vi "MakeEngine.vi"(8 "error in (no error)":errorcluster, 11 "ClassicType in":refnum<class "ClassicType.lvclass">) -> (0 "error out":errorcluster, 3 "ClassicType out":refnum<class "ClassicType.lvclass">)   [LabVIEW 2021, in "ClassicType.lvclass"]
uses:
  ClassicType.lvclass
  C:/Users/chrismadlax/Documents/LabVIEW Data/Project/OOP/GeneralCar/GeneralCar.lvclass
  GeneralCar/GeneralCar.lvclass/GeneralCar.ctl
  GeneralCar/GeneralCar.lvclass
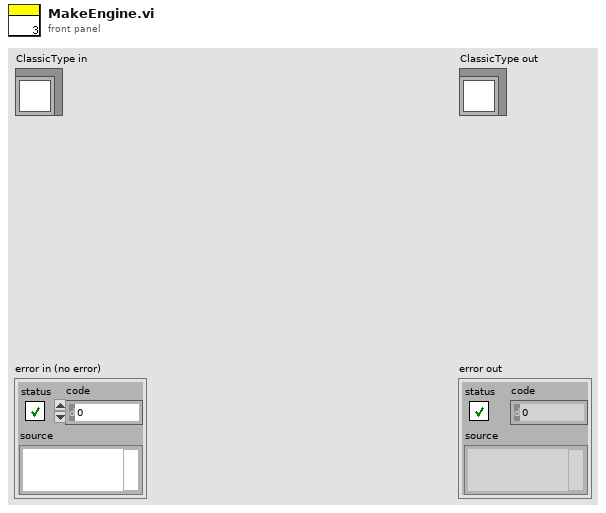
[diagram p1: front panel]
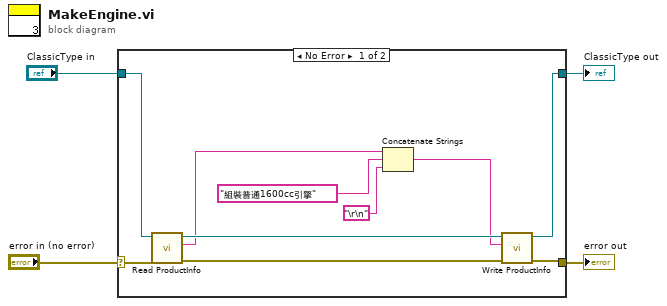
[diagram p0: block diagram]
diagram:
  n1 = case shown="No Error" "error in (no error)" {
    selector: "error in (no error)" -> [w7 w16]
    tunnel: [w6 w16] -> w4
    tunnel: [w5 w15] -> w3
    tunnel: "ClassicType in" -> [w8 w15]
    frame No Error {
      n2 = call "Read ProductInfo.vi"("error in (no error)"=w7, "GeneralCar in"=w8) -> ("error out"=w14:errorcluster, "ProductInfo"=w10:string, "GeneralCar out"=w13:refnum<class "ClassicType.lvclass">)  [unwired: 7 in]
      n3 = Concatenate Strings(w10, "組裝普通1600cc引擎" ("string"), "\r\n") -> (w9:string)
      n4 = call "Write ProductInfo.vi"("error in (no error)"=w14, "ProductInfo"=w9, "GeneralCar in"=w13) -> ("error out"=w6:errorcluster, "GeneralCar out"=w5:refnum<class "ClassicType.lvclass">)  [unwired: 7 in]
    }
    frame Error {
    }
  }
  "error out" <- w4
  "ClassicType out" <- w3
